vi "get_authorization.vi"(8 "error in (no error)":errorcluster) -> (0 "error out":errorcluster, 2 "expire":timestamp, 3 "authorization":string)   [LabVIEW 2015, in "lv-dropbox.lvlib"]
uses:
  lv-dropbox.lvlib
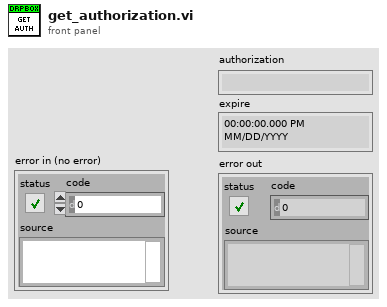
[diagram p1: front panel]
types:
  T1 = typedef "lv-dropbox.lvlib/authorization.ctl" = cluster{"authorization":string, "expire":timestamp}
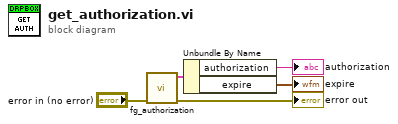
[diagram p0: block diagram]
diagram:
  n1 = call "fg_authorization.vi"("error in (no error)"="error in (no error)") -> ("error out"=→"error out":errorcluster, "authorization out"=w3:T1)  [unwired: 9 in]
  n2 = Unbundle By Name(w3) -> ("authorization"=→"authorization":string, "expire"=→"expire":timestamp)
